vi "Message selection.vi"(8 "error in (no error)":errorcluster, 9 "Amount":dbl, 10 "state":T1, 11 "Message type":string) -> (0 "error out":errorcluster, 3 "Msg":string)   [LabVIEW 2019, in "SubVI.lvlib"]
uses:
  ATM/controls/Message Type.ctl
  SubVI.lvlib
panel:
  # "All Messages"
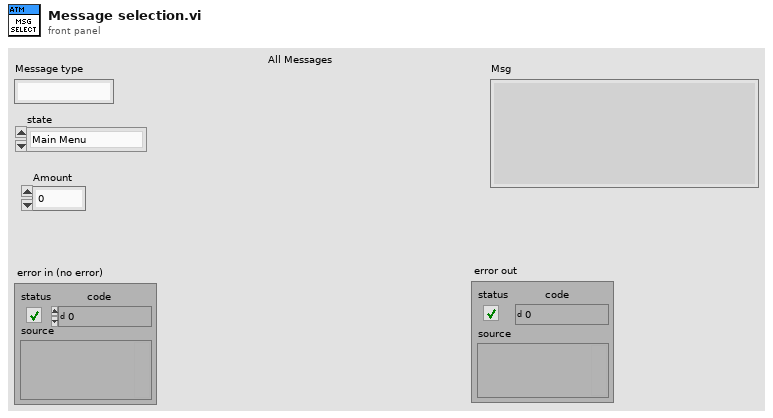
[diagram p1: front panel]
types:
  T1 = typedef "Message Type.ctl" = enum16{"Main Menu", "Balance", "Withdrawal Complete", "Deposit Complete", "Welcome", "Account", "Session", "Deposit", "Withdraw", "Failed"}
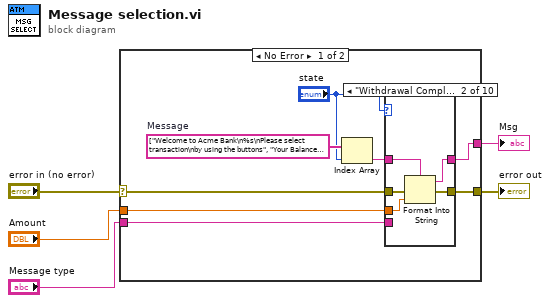
[diagram p0: block diagram]
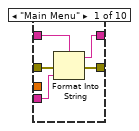
[diagram p2: hidden frame]
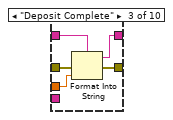
[diagram p3: hidden frame]
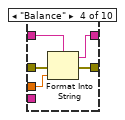
[diagram p4: hidden frame]
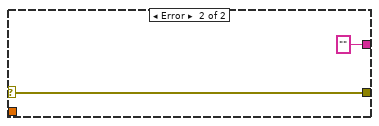
[diagram p11: hidden frame]
diagram:
  n1 = case shown="No Error" "error in (no error)" {
    selector: "error in (no error)" -> [w10 w47]
    tunnel: [w9 w47] -> w4
    tunnel: "Message type" -> [w13 _]
    tunnel: "Amount" -> [w12 _]
    tunnel: [w11 ""] -> w1
    frame No Error {
      w8 = string[] ["Welcome to Acme Bank\n%s\nPlease select transaction\nby using the buttons", "Your Balance Is:\n$ %d", "$ %d Withdrawn", "$ %d Deposited", "Welcome to Acme Bank.\nPlease insert your card\nand enter your account\nnumber in the User Input.\nPress Enter (E) when done.", "Account Information Incorrect\nPlease Re-Enter Account Number.\nPress Enter (E) when done\n", "Your session has been terminated\ndue to inactivity or menu selection.\nPlease take your card\nGoodbye!", "Please enter amount to deposit and press \nEnter (E) when done", "Please enter amount to withdraw and press \nEnter (E) when done", "Insufficient funds in account\nPlease check your balance\nand try again"]  # Message
      n2 = Index Array(array=w8, index="state") -> (element=w6:string)
      n3 = case shown="\"Withdrawal Complete\"" "state" {
        tunnel: w13 -> [w17 _ _ _ _ _ _ _ _ _]
        tunnel: w12 -> [_ w22 w27 w32 _ _ _ _ _ _]
        tunnel: [w18 w23 w28 w33 w35 w37 w39 w41 w43 w45] -> w11
        tunnel: w10 -> [w16 w21 w26 w31 w34 w36 w38 w40 w42 w44]
        tunnel: [w15 w20 w25 w30 w34 w36 w38 w40 w42 w44] -> w9
        tunnel: w6 -> [w14 w19 w24 w29 w35 w37 w39 w41 w43 w45]
        frame "Main Menu" {
          n4 = Format Into String(format string=w14, error in=w16, w17) -> (resulting string=w18:string, error out=w15:errorcluster)  [unwired: 1 in]
        }
        frame "Withdrawal Complete" {
          n5 = Format Into String(format string=w19, error in=w21, w22) -> (resulting string=w23:string, error out=w20:errorcluster)  [unwired: 1 in]
        }
        frame "Deposit Complete" {
          n6 = Format Into String(format string=w24, error in=w26, w27) -> (resulting string=w28:string, error out=w25:errorcluster)  [unwired: 1 in]
        }
        frame "Balance" {
          n7 = Format Into String(format string=w29, error in=w31, w32) -> (resulting string=w33:string, error out=w30:errorcluster)  [unwired: 1 in]
        }
        frame "Welcome" {
        }
        frame "Account" {
        }
        frame "Session" {
        }
        frame "Deposit" {
        }
        frame "Withdraw" {
        }
        frame "Failed" {
        }
      }
    }
    frame Error {
    }
  }
  "Msg" <- w1
  "error out" <- w4
